vi "Configure Spurious Emission (Time Domain Setup).vi"(0 "VISA resource name":refnum<visa-resource-name>, 1 "Spurious Detection Mode":i32[](array[ring]) items=["Positive", "Sample", "RMS"], 5 "Spurious Auto Resolution Bandwidth":i32[](array[ring]) items=["Off", "On"], 7 "Spurious Resolution Bandwidth":i32[](array[ring]) items=["30 Hz", "100 Hz", "300 Hz", "1 kHz", "3 kHz", "10 kHz", "30 kHz", "100 kHz", "300 kHz", "1 MHz", "3 MHz", "50 kHz", "5 MHz", "10 MHz", "20 MHz", "31.25MHz"], 9 "Spurious Auto Video Bandwidth":i32[](array[ring]) items=["Off", "On"], 11 "error in (no error)":errorcluster, 12 "Spurious Video Bandwidth":i32[](array[ring]) items=["Off", "1 Hz", "3 Hz", "10 Hz", "30 Hz", "100 Hz", "300 Hz", "1 kHz", "3 kHz", "10 kHz", "30 kHz", "100 kHz", "300 kHz", "1 MHz", "3 MHz", "10 MHz", "5 kHz"], 13 "Spurious Sweep Time":dbl[](array[numeric]) min=1e-06 max=1000.0) -> (4 "VISA resource name out":refnum<visa-resource-name>, 15 "error out":errorcluster)   [LabVIEW 2020, in "Anritsu Signal Analyzer Series.lvlib"]
doc: "Configures the time domain for Spurious Emission measurement."
uses:
  Anritsu Signal Analyzer Series.lvlib
panel:
  # "s"
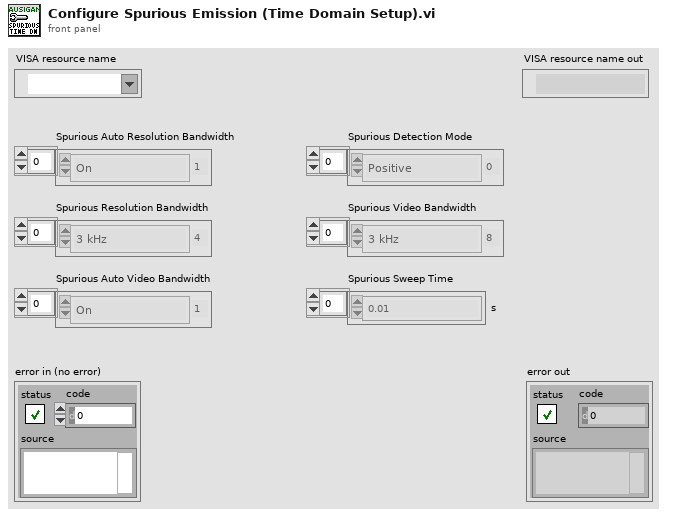
[diagram p1: front panel]
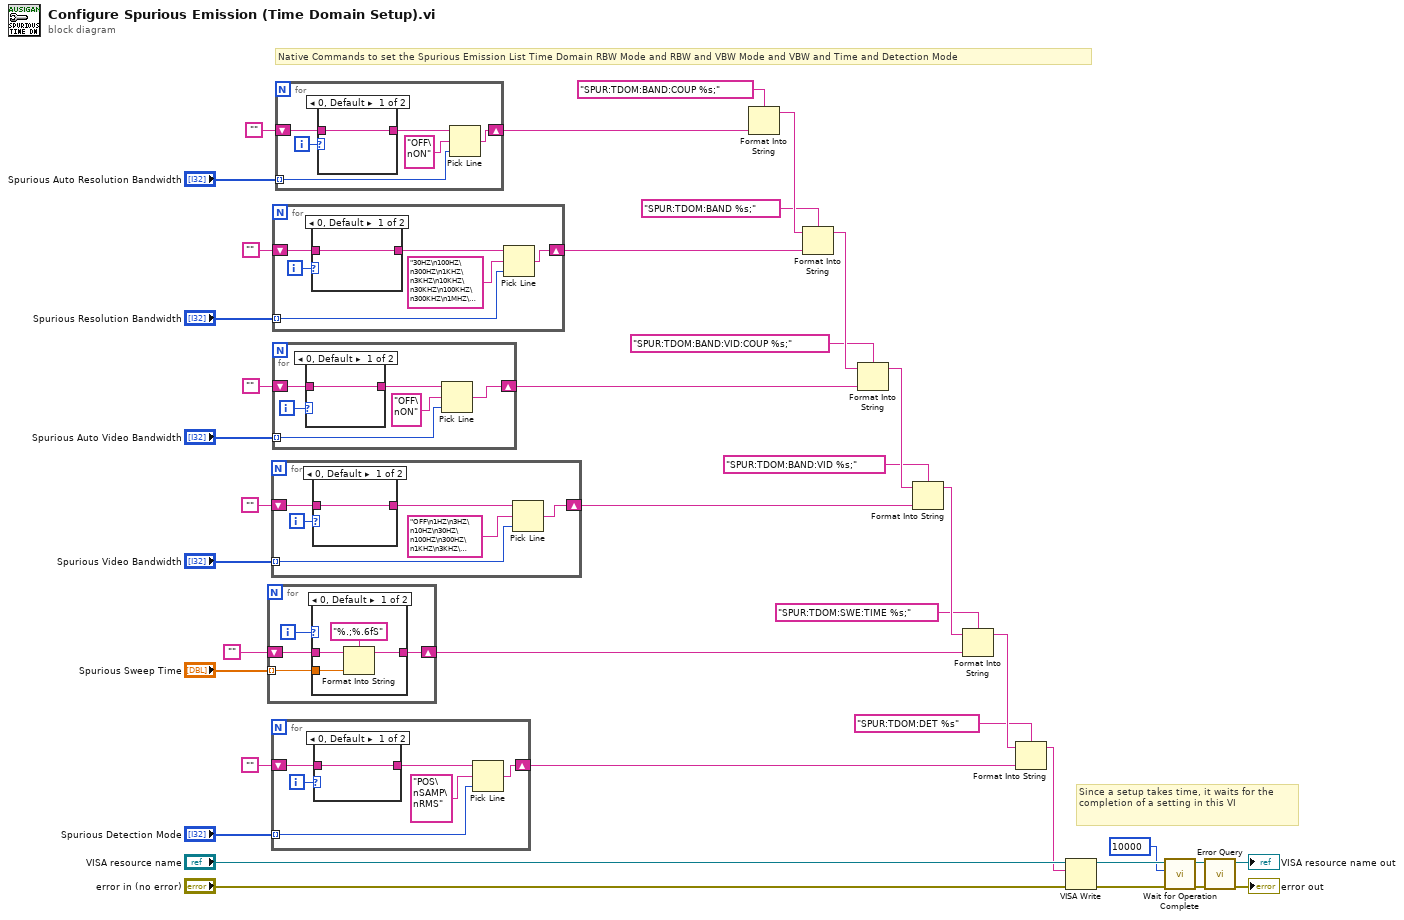
[diagram p0: block diagram]
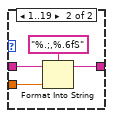
[diagram p2: hidden frame]
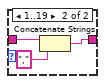
[diagram p3: hidden frame]
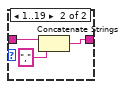
[diagram p4: hidden frame]
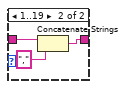
[diagram p5: hidden frame]
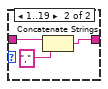
[diagram p6: hidden frame]
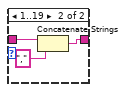
[diagram p7: hidden frame]
diagram:
  # "Since a setup takes time, it waits for the completion of a setting in this VI"
  # "Native Commands to set the Spurious Emission List Time Domain RBW Mode and RBW and VBW Mode and VBW and Time and Detection Mode"
  n1 = for {
    shift-right: [w40] -> w7
    shift-left: "" -> [w42]
    tunnel: "Spurious Sweep Time" -> [w41] mode=indexing
    i -> [w43]
    n2 = case shown="0, Default" w43 {
      tunnel: w42 -> [w46 w49]
      tunnel: [w44 w48] -> w40
      tunnel: w41 -> [w45 w50]
      frame 0, Default {
        n3 = Format Into String(format string="%.;%.6fS" ("string"), initial string=w46, w45) -> (resulting string=w44:string)  [unwired: 1 in, 1 out]
      }
      frame 1..19 {
        n4 = Format Into String(format string="%.;,%.6fS" ("string"), initial string=w49, w50) -> (resulting string=w48:string)  [unwired: 1 in, 1 out]
      }
    }
  }
  n5 = for {
    shift-right: [w53] -> w18
    shift-left: "" -> [w56]
    tunnel: "Spurious Video Bandwidth" -> [w52] mode=indexing
    i -> [w57]
    n6 = case shown="0, Default" w57 {
      tunnel: w56 -> [w58 w61]
      tunnel: [w58 w59] -> w54
      frame 0, Default {
      }
      frame 1..19 {
        n7 = Concatenate Strings(w61, "," ("string")) -> (w59:string)
      }
    }
    n8 = Pick Line(string ("")=w54, multi-line string="OFF\n1HZ\n3HZ\n10HZ\n30HZ\n100HZ\n300HZ\n1KHZ\n3KHZ\n10KHZ\n30KHZ\n100KHZ\n300KHZ\n1MHZ\n3MHZ\n5MHZ\n10MHZ\n5KHZ" ("複数行文字列"), line index=w52) -> (output string=w53:string)
  }
  n9 = for {
    shift-right: [w63] -> w12
    shift-left: "" -> [w66]
    tunnel: "Spurious Detection Mode" -> [w62] mode=indexing
    i -> [w67]
    n10 = case shown="0, Default" w67 {
      tunnel: w66 -> [w68 w71]
      tunnel: [w68 w69] -> w64
      frame 0, Default {
      }
      frame 1..19 {
        n11 = Concatenate Strings(w71, "," ("string")) -> (w69:string)
      }
    }
    n12 = Pick Line(string ("")=w64, multi-line string="POS\nSAMP\nRMS" ("複数行文字列"), line index=w62) -> (output string=w63:string)
  }
  n13 = for {
    shift-right: [w73] -> w26
    shift-left: "" -> [w76]
    tunnel: "Spurious Resolution Bandwidth" -> [w72] mode=indexing
    i -> [w77]
    n14 = case shown="0, Default" w77 {
      tunnel: w76 -> [w78 w81]
      tunnel: [w78 w79] -> w74
      frame 0, Default {
      }
      frame 1..19 {
        n15 = Concatenate Strings(w81, "," ("string")) -> (w79:string)
      }
    }
    n16 = Pick Line(string ("")=w74, multi-line string="30HZ\n100HZ\n300HZ\n1KHZ\n3KHZ\n10KHZ\n30KHZ\n100KHZ\n300KHZ\n1MHZ\n3MHZ\n50KHZ\n5MHZ\n10MHZ\n20MHZ\n31.25MHZ" ("複数行文字列"), line index=w72) -> (output string=w73:string)
  }
  n17 = for {
    shift-right: [w82] -> w22
    shift-left: "" -> [w86]
    tunnel: "Spurious Auto Video Bandwidth" -> [w84] mode=indexing
    i -> [w87]
    n18 = case shown="0, Default" w87 {
      tunnel: w86 -> [w88 w91]
      tunnel: [w88 w89] -> w83
      frame 0, Default {
      }
      frame 1..19 {
        n19 = Concatenate Strings(w91, "," ("string")) -> (w89:string)
      }
    }
    n20 = Pick Line(string ("")=w83, multi-line string="OFF\nON" ("複数行文字列"), line index=w84) -> (output string=w82:string)
  }
  n21 = for {
    shift-right: [w92] -> w29
    shift-left: "" -> [w96]
    tunnel: "Spurious Auto Resolution Bandwidth" -> [w93] mode=indexing
    i -> [w97]
    n22 = case shown="0, Default" w97 {
      tunnel: w96 -> [w98 w101]
      tunnel: [w98 w99] -> w94
      frame 0, Default {
      }
      frame 1..19 {
        n23 = Concatenate Strings(w101, "," ("string")) -> (w99:string)
      }
    }
    n24 = Pick Line(string ("")=w94, multi-line string="OFF\nON" ("複数行文字列"), line index=w93) -> (output string=w92:string)
  }
  n25 = Format Into String(format string="SPUR:TDOM:BAND:COUP %s;" ("_CommandSet"), w29) -> (resulting string=w25:string)  [unwired: 2 in, 1 out]
  n26 = Format Into String(format string="SPUR:TDOM:BAND %s;" ("_CommandSet"), initial string=w25, w26) -> (resulting string=w21:string)  [unwired: 1 in, 1 out]
  n27 = Format Into String(format string="SPUR:TDOM:BAND:VID:COUP %s;" ("_CommandSet"), initial string=w21, w22) -> (resulting string=w17:string)  [unwired: 1 in, 1 out]
  n28 = Format Into String(format string="SPUR:TDOM:BAND:VID %s;" ("_CommandSet"), initial string=w17, w18) -> (resulting string=w15:string)  [unwired: 1 in, 1 out]
  n29 = Format Into String(format string="SPUR:TDOM:SWE:TIME %s;" ("_CommandSet"), initial string=w15, w7) -> (resulting string=w11:string)  [unwired: 1 in, 1 out]
  n30 = Format Into String(format string="SPUR:TDOM:DET %s" ("_CommandSet"), initial string=w11, w12) -> (resulting string=w9:string)  [unwired: 1 in, 1 out]
  n31 = VISA Write(VISA resource name="VISA resource name", write buffer=w9, error in (no error)="error in (no error)") -> (VISA resource name out=w4:refnum<visa-resource-name>, error out=w3:errorcluster)  [unwired: 1 out]
  n32 = call "Wait for Operation Complete.vi"("error in (no error)"=w3, "Maximum Time (10000mSec)"=10000, "VISA resource name"=w4) -> ("error out"=w5:errorcluster, "VISA resource name out"=w6:refnum<visa-resource-name>)  [unwired: 7 in]
  n33 = call "Error Query.vi"("error in (no error)"=w5, "VISA resource name"=w6) -> ("error out"=→"error out":errorcluster, "VISA resource name out"=→"VISA resource name out":refnum<visa-resource-name>)  [unwired: 6 in, 2 out]
